vi "Export Intensity Graph Image to Notebook.vi"(8 "Error In":errorcluster, 9 "Intensity Graph Ref":refnum<vi>, 11 "Notebook Q":refnum<queue>) -> (0 "Error Out":errorcluster)   [LabVIEW 2021, in "Notebook.lvlib"]
uses:
  Notebook.lvlib
  Notebook Action Q Element.ctl
  Notebook Action List.ctl
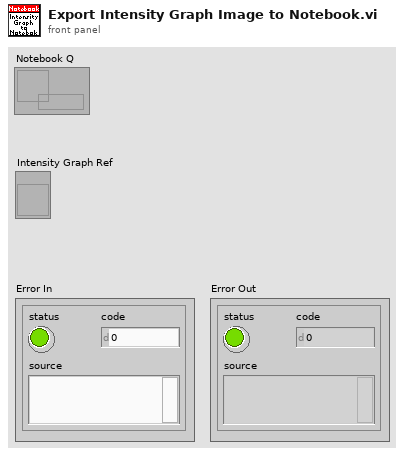
[diagram p1: front panel]
types:
  T1 = typedef "Notebook.lvlib/Notebook Action Q Element.ctl" = cluster{"Action":T2, "Variant":variant}
  T2 = typedef "Notebook.lvlib/Notebook Action List.ctl" = enum16{"Idle", "Init", "Check Content Change", "User added content", "Program added text", "Program added Picture ", "Save Notebook", "Quit", "Open", "Close", "Update Window Title"}
  T3 = typedef "imagedata.ctl" = cluster{"image type":i32, "image depth":i32, "image":u8[], "mask":u8[], "colors":u32[], "Rectangle":cluster{"left":i16, "top":i16, "right":i16, "bottom":i16}}
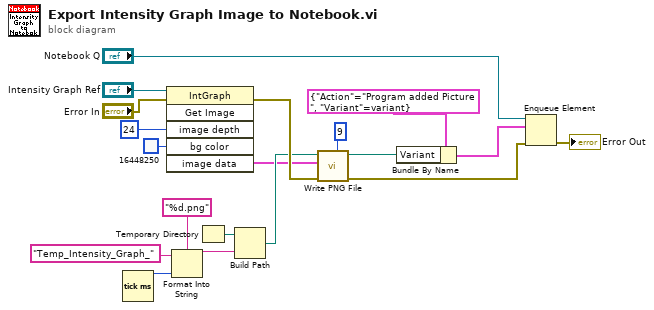
[diagram p0: block diagram]
diagram:
  n1 = Tick Count (ms)() -> (millisecond timer value=w10:u32)
  n2 = invoke on="Invoke Node" class="IntGraph" method="Get Image"(reference="Intensity Graph Ref", error in="Error In", "image depth"=24 ("Image Depth"), "bg color"=u32 16448250 ("Background Color")) -> (error out=w8:errorcluster, "image data"=w6:T3)  [unwired: 2 in, 4 out]
  n3 = Format Into String(format string="%d.png", initial string="Temp_Intensity_Graph_", w10) -> (resulting string=w11:string)  [unwired: 1 in, 1 out]
  n4 = Temporary Directory() -> (w9:path)
  n5 = Build Path(base path=w9, name or relative path=w11) -> (appended path=w7:path)
  n6 = call <vilib>:"Write PNG File.vi"("compression (default)"=9, "error in (no error)"=w8, "image data"=w6, "path to PNG file"=w7) -> ("error out"=w2:errorcluster, "path"=w13:path)  [unwired: 6 in]
  n7 = Bundle By Name(cluster=T1 {"Action"=enum."Program added Picture ", "Variant"=variant} ("element"), "Variant"=w13) -> (w4:T1)
  n8 = Enqueue Element(queue="Notebook Q", element=w4, error in (no error)=w2) -> (error out=→"Error Out":errorcluster)  [unwired: 1 in, 2 out]
